vi "ToMatlabType.vi"(11 "Value":variant) -> (0 "IsNumeric":bool, 1 "Type":T3, 2 "Name":string, 3 "MatlabType":T2, 4 "Container Type (Labview Value type)":T1)   [LabVIEW 2017]
uses:
  <vilib>/Utility/Data Type/Type Definitions/Data Type.ctl
  Types/MatlabDataType.ctl
  Types/MatlabDataContainerType.ctl
  <vilib>/Utility/Data Type/NI_Data Type.lvlib
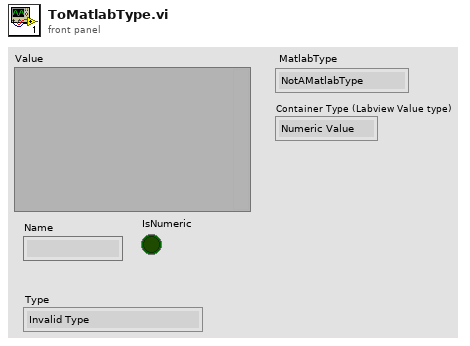
[diagram p1: front panel]
types:
  T1 = typedef "MatlabDataContainerType.ctl" = enum16{"Numeric Value", "Numeric Array", "Waveform"}
  T2 = typedef "MatlabDataType.ctl" = enum16{"NotAMatlabType", "Real", "Complex", "String", "Boolean"}
  T3 = typedef "NI_Data Type.lvlib/Data Type.ctl" = enum8{"Invalid Type", "Void", "I8", "I16", "I32", "I64", "U8", "U16", "U32", "U64", "Single Float", "Double Float", "Extended Float", "Single Complex", "Double Complex", "Extended Complex", "Enum U8", "Enum U16", "Enum U32", "Enum U64", "Single Float With Unit", "Double Float With Unit", "Extended Float With Unit", "Single Complex with Unit", "Double Complex with Unit", "Extended Complex with Unit", "Boolean", "String", "Path", "Picture", "Tag", "Array", "Cluster", "Variant", "LV Variant", "Waveform", "Timestamp", "Digital Waveform", "Digital Data", "ExpressData", "Refnum", "External Data", "VI", "Poly VI", "LabVIEW Class Instance", "Fixed Point"}
  T4 = typedef "Waveform Subtype Enum__ogtk.ctl" = enum8{"<Not a Waveform Type>", "0x01", "Analog 16-bit signed", "Analog Double-Precision", "0x04", "Analog Single Precision", "Timestamp", "Digital Data", "Digital Waveform", "Dynamic Data", "Analog Extended-Precision", "Analog 8-bit unsigned", "Analog 16-bit unsigned", "Analog 32-bit unsigned", "Analog 8-bit signed", "Analog 32-bit signed", "Analog Complex Single-Precision", "Analog Complex Double-Precision", "Analog Complex Extended Precision", "Analog 64-bit signed", "Analog 64-bit unsigned"}
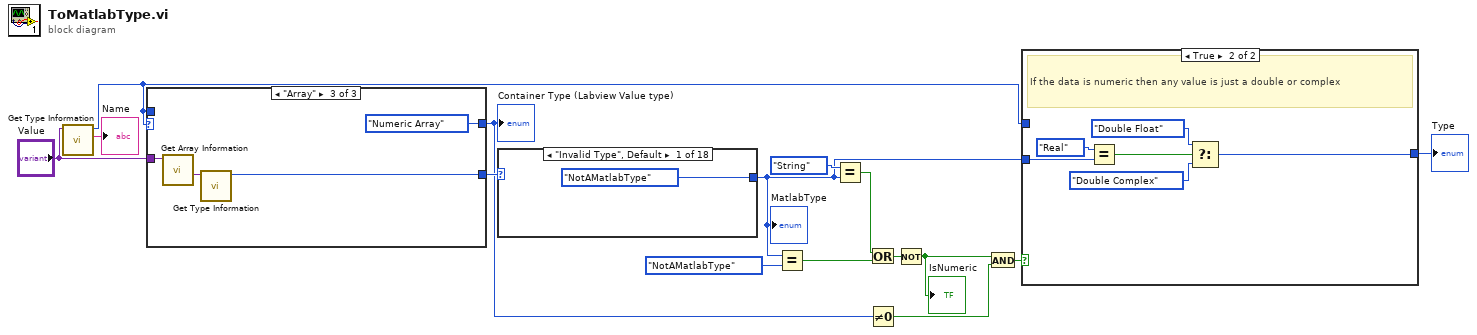
[diagram p0: block diagram]
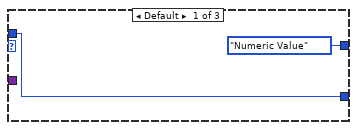
[diagram p3: hidden frame]
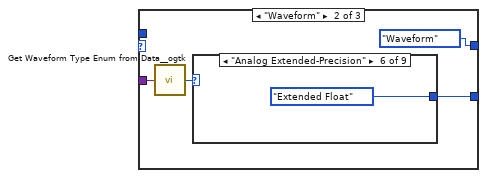
[diagram p4: hidden frame]
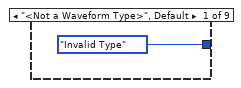
[diagram p5: hidden frame]
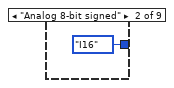
[diagram p6: hidden frame]
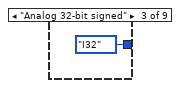
[diagram p7: hidden frame]
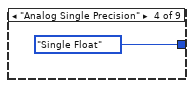
[diagram p8: hidden frame]
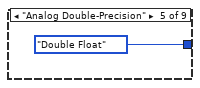
[diagram p9: hidden frame]
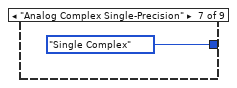
[diagram p10: hidden frame]
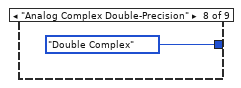
[diagram p11: hidden frame]
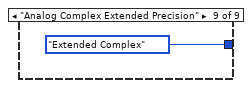
[diagram p12: hidden frame]
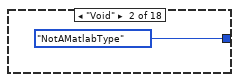
[diagram p13: hidden frame]
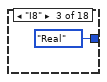
[diagram p14: hidden frame]
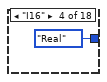
[diagram p15: hidden frame]
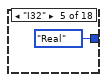
[diagram p16: hidden frame]
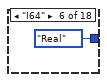
[diagram p17: hidden frame]
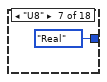
[diagram p18: hidden frame]
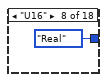
[diagram p19: hidden frame]
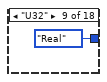
[diagram p20: hidden frame]
diagram:
  n1 = call <vilib>:"Get Type Information.vi"("Variant"="Value") -> ("Name"=→"Name":string, "Type"=w7:T3)  [unwired: 6 in, 3 out]
  n2 = case shown="\"Array\"" w7 {
    tunnel: "Value" -> [_ w21 w34]
    tunnel: [w17 w19 w32] -> w14
    tunnel: w7 -> [w17 _ _]
    tunnel: [MatlabDataContainerType."Numeric Value" MatlabDataContainerType."Waveform" MatlabDataContainerType."Numeric Array"] -> w2
    frame Default {
    }
    frame "Waveform" {
      n3 = call <userlib>:"Get Waveform Type Enum from Data__ogtk.vi"("Data"=w21) -> ("Waveform Subtype Enum"=w20:T4)  [unwired: 4 in]
      n4 = case shown="\"Analog Extended-Precision\"" w20 {
        tunnel: [Data_Type."Invalid Type" ("Type") Data_Type."I16" ("Type") Data_Type."I32" ("Type") Data_Type."Single Float" ("Type") Data_Type."Double Float" ("Type") Data_Type."Extended Float" ("Type") Data_Type."Single Complex" ("Type") Data_Type."Double Complex" ("Type") Data_Type."Extended Complex" ("Type")] -> w19
        frame "<Not a Waveform Type>", Default {
        }
        frame "Analog 8-bit signed" {
        }
        frame "Analog 32-bit signed" {
        }
        frame "Analog Single Precision" {
        }
        frame "Analog Double-Precision" {
        }
        frame "Analog Extended-Precision" {
        }
        frame "Analog Complex Single-Precision" {
        }
        frame "Analog Complex Double-Precision" {
        }
        frame "Analog Complex Extended Precision" {
        }
      }
    }
    frame "Array" {
      n5 = call <vilib>:"Get Array Information.vi"("Variant"=w34) -> ("Array Element Data Type"=w33:variant)  [unwired: 7 in, 3 out]
      n6 = call <vilib>:"Get Type Information.vi"("Variant"=w33) -> ("Type"=w32:T3)  [unwired: 6 in, 4 out]
    }
  }
  "Container Type (Labview Value type)" <- w2
  n7 = case shown="\"Invalid Type\", Default" w14 {
    tunnel: [MatlabDataType."NotAMatlabType" ("MatlabType") MatlabDataType."NotAMatlabType" ("MatlabType") MatlabDataType."Real" ("MatlabType") MatlabDataType."Real" ("MatlabType") MatlabDataType."Real" ("MatlabType") MatlabDataType."Real" ("MatlabType") MatlabDataType."Real" ("MatlabType") MatlabDataType."Real" ("MatlabType") MatlabDataType."Real" ("MatlabType") MatlabDataType."Real" ("MatlabType") MatlabDataType."Real" ("MatlabType") MatlabDataType."Real" ("MatlabType") MatlabDataType."Real" ("MatlabType") MatlabDataType."Complex" ("MatlabType") MatlabDataType."Complex" ("MatlabType") MatlabDataType."Complex" ("MatlabType") MatlabDataType."String" ("MatlabType") MatlabDataType."Boolean" ("MatlabType")] -> w3
    frame "Invalid Type", Default {
    }
    frame "Void" {
    }
    frame "I8" {
    }
    frame "I16" {
    }
    frame "I32" {
    }
    frame "I64" {
    }
    frame "U8" {
    }
    frame "U16" {
    }
    frame "U32" {
    }
    frame "U64" {
    }
    frame "Single Float" {
    }
    frame "Double Float" {
    }
    frame "Extended Float" {
    }
    frame "Single Complex" {
    }
    frame "Double Complex" {
    }
    frame "Extended Complex" {
    }
    frame "String" {
    }
    frame "Boolean" {
    }
  }
  "MatlabType" <- w3
  n8 = Equal?(x=w3, y=MatlabDataType."NotAMatlabType" ("MatlabType")) -> (x = y?=w11:bool)
  n9 = Equal?(x=MatlabDataType."String" ("MatlabType"), y=w3) -> (x = y?=w12:bool)
  n10 = Or(x=w12, y=w11) -> (x .or. y?=w10:bool)
  n11 = Not Equal To 0?(x=w2) -> (x != 0?=w1:bool)
  n12 = Not(x=w10) -> (.not. x?=w5:bool)
  "IsNumeric" <- w5
  n13 = And(x=w5, y=w1) -> (x .and. y?=w4:bool)
  n14 = case shown="True" w4 {
    tunnel: w7 -> [w53 _]
    tunnel: [w53 w54] -> w6
    tunnel: w3 -> [_ w57]
    frame False {
    }
    frame True {
      # "If the data is numeric then any value is just a double or complex"
      n15 = Equal?(x=MatlabDataType."Real" ("MatlabType"), y=w57) -> (x = y?=w59:bool)
      n16 = Select(t=Data_Type."Double Float" ("Type"), s=w59, f=Data_Type."Double Complex" ("Type")) -> (s? t:f=w54:T3)
    }
  }
  "Type" <- w6
